vi "PlaneFit_flt.vi"(6 "Planing y/n?":bool, 7 "Reset Clicks":bool, 8 "Y PEN":dbl, 9 "Z":dbl, 10 "Nano Z":dbl, 11 "X":dbl) -> (2 "Plane Height (m)":dbl, 3 "Clicks":i32, 5 "Planing Done?":bool)   [LabVIEW 2017]
uses:
  Program Files/National Instruments/LabVIEW 2019/user.lib/HapticSTM/HapticSTM.lvlib
  GlobalClicksHeight_flt.vi
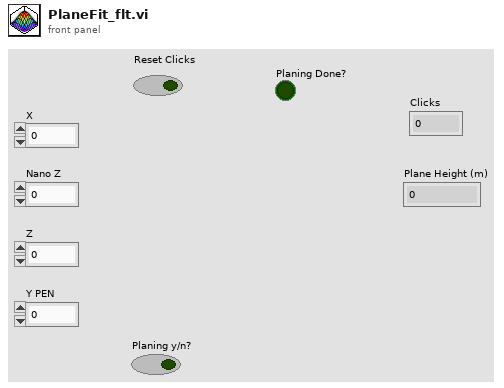
[diagram p1: front panel]
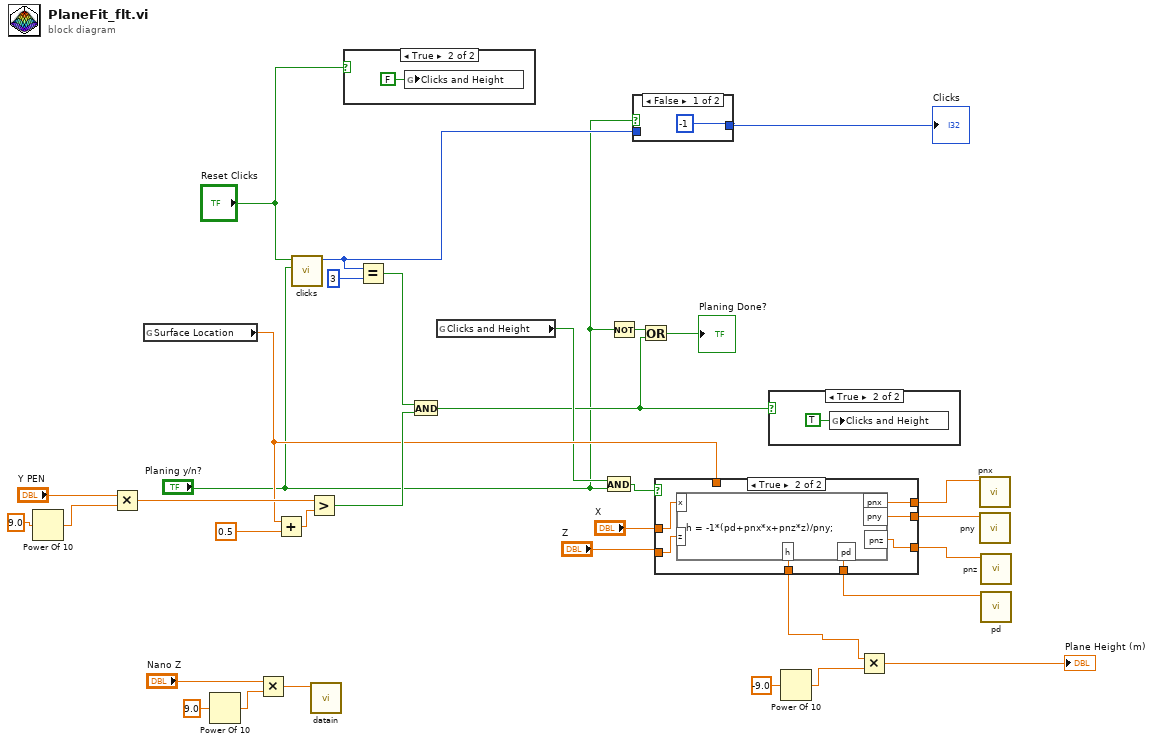
[diagram p0: block diagram]
diagram:
  n1 = Power Of 10(x=9.0) -> (10^x=w22:dbl)
  n2 = Multiply(x="Y PEN", y=w22) -> (x*y=w19:dbl)
  n3 = global read "GlobalClicksHeight_flt.vi" "Surface Location"() -> (w12:dbl)
  n4 = Power Of 10(x=9.0) -> (10^x=w18:dbl)
  n5 = Multiply(x="Nano Z", y=w18) -> (x*y=w14:dbl)
  n6 = Add(x=w12, y=0.5) -> (x+y=w24:dbl)
  n7 = call "clicks.vi"("planing"="Planing y/n?", "reset"="Reset Clicks") -> ("function return"=w9:i32)  [unwired: 9 in]
  n8 = Greater?(x=w19, y=w24) -> (0:w25:bool)
  n9 = call "datain.vi"("output"=w14) -> ()  [unwired: 11 in]
  n10 = case shown="True" "Reset Clicks" {
    frame False {
    }
    frame True {
      n11 = global write "GlobalClicksHeight_flt.vi" "Clicks and Height"(FALSE ("Clicks and Height")) -> ()
    }
  }
  n12 = Equal?(x=w9, y=3) -> (x = y?=w26:bool)
  n13 = And(x=w26, y=w25) -> (x .and. y?=w7:bool)
  n14 = global read "GlobalClicksHeight_flt.vi" "Clicks and Height"() -> (w11:bool)
  n15 = And(x=w11, y="Planing y/n?") -> (x .and. y?=w10:bool)
  n16 = Not(x="Planing y/n?") -> (.not. x?=w5:bool)
  n17 = case shown="False" "Planing y/n?" {
    tunnel: w9 -> [_ w36]
    tunnel: [-1 ("function return") w36] -> w8
    frame False {
    }
    frame True {
    }
  }
  "Clicks" <- w8
  n18 = Or(x=w5, y=w7) -> (x .or. y?=→"Planing Done?":bool)
  n19 = case shown="True" w7 {
    frame False {
    }
    frame True {
      n20 = global write "GlobalClicksHeight_flt.vi" "Clicks and Height"(TRUE ("Clicks and Height")) -> ()
    }
  }
  n21 = Power Of 10(x=-9.0) -> (10^x=w28:dbl)
  n22 = call "pnx.vi"() -> ("function return"=w30:dbl)  [unwired: 11 in]
  n23 = call "pny.vi"() -> ("function return"=w29:dbl)  [unwired: 11 in]
  n24 = call "pnz.vi"() -> ("function return"=w33:dbl)  [unwired: 11 in]
  n25 = call "pd.vi"() -> ("function return"=w32:dbl)  [unwired: 11 in]
  n26 = case shown="True" w10 {
    tunnel: "X" -> [_ w45]
    tunnel: w30 -> [_ w43]
    tunnel: w29 -> [_ w42]
    tunnel: w33 -> [_ w41]
    tunnel: w32 -> [_ w40]
    tunnel: "Z" -> [_ w44]
    tunnel: [w38 w39] -> w1
    tunnel: w12 -> [w38 _]
    frame False {
    }
    frame True {
      n27 = formula code="h = -1*(pd+pnx*x+pnz*z)/pny;"("x"=w45, "z"=w44, "pnx"=w43, "pnz"=w41, "pd"=w40, "pny"=w42) -> ("h"=w39:dbl)
    }
  }
  n28 = Multiply(x=w1, y=w28) -> (x*y=→"Plane Height (m)":dbl)
